vi "HV_Manual_Control_sethv_Path.vi"() -> (3 "sethv filepath":path)   [LabVIEW 2018]
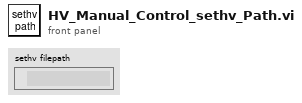
[diagram p1: front panel]
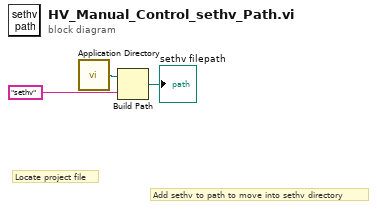
[diagram p0: block diagram]
diagram:
  # "Add sethv to path to move into sethv directory"
  # "Locate project file"
  n1 = call <vilib>:"Application Directory.vi"() -> ("Application Directory"=w3:path)
  n2 = Build Path(base path=w3, name or relative path="sethv") -> (appended path=→"sethv filepath":path)
